vi "RP-VOA CALIBRATION FIT.vi"(2 "error in (no error)":errorcluster, 4 "file path":path) -> (0 "error out":errorcluster, 1 "Calibration array":dbl[](array[numeric]))   [LabVIEW 2021]
uses:
  <vilib>/Utility/file.llb/Read Delimited Spreadsheet (DBL).vi
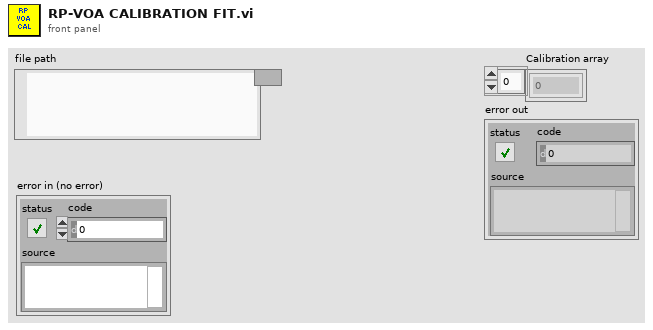
[diagram p1: front panel]
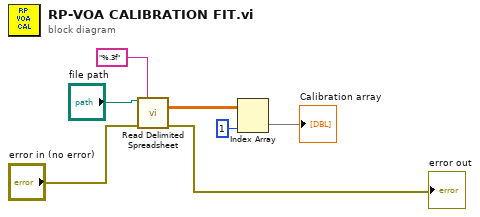
[diagram p0: block diagram]
diagram:
  n1 = call-poly <vilib>:"Read Delimited Spreadsheet.vi"("file path (dialog if empty)"="file path", "format (%.3f)"="%.3f", "error in (no error)"="error in (no error)") -> ("all rows"=w6:dbl[][], "error out"=→"error out":errorcluster)  [unwired: 7 in, 4 out]
  n2 = Index Array(array=w6, index (col)=1 ("disabled index (col)")) -> (element=→"Calibration array":dbl[])  [unwired: 1 in]
